vi "Configure Measurements.vi"   [LabVIEW 2015, in "Voltech PM1000+.lvlib"]
uses:
  <instrlib>/Voltech PM1000+/Voltech PM1000+.lvlib
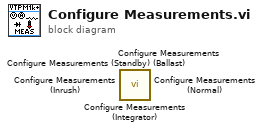
[diagram p0: block diagram]
diagram:
  n1 = call <instrlib>:"Configure Measurements (Integrator).vi"() -> ()  [unwired: 10 in, 2 out]
  n2 = call <instrlib>:"Configure Measurements (Ballast).vi"() -> ()  [unwired: 10 in, 2 out]
  n3 = call <instrlib>:"Configure Measurements (Inrush).vi"() -> ()  [unwired: 10 in, 2 out]
  n4 = call <instrlib>:"Configure Measurements (Normal).vi"() -> ()  [unwired: 10 in, 2 out]
  n5 = call <instrlib>:"Configure Measurements (Standby).vi"() -> ()  [unwired: 10 in, 2 out]
